vi "SteuerungWaermepumpe - 10.0117_ohne Keithley.vi"() -> ()   [LabVIEW 2015]
uses:
  <vilib>/DAQmx/read.llb/DAQmx Read (Analog 1D Wfm NChan NSamp).vi
  <vilib>/DAQmx/write.llb/DAQmx Write (Analog 1D Wfm NChan 1Samp).vi
  <vilib>/MakerHub/LINX/Public/Peripherals/Digital/Digital Write N Chans.vi
  <vilib>/MakerHub/LINX/Private/Local IO/LinxDigitalWrite.vi
  <vilib>/MakerHub/LINX/Public/Utilities/Check Channel.vi
  <vilib>/MakerHub/LINX/Private/Utilties/Generate Error.vi
  <vilib>/DAQmx/miscellaneous.llb/DAQmx Fill In Error Info.vi
  <vilib>/Utility/file.llb/Read Delimited Spreadsheet (DBL).vi
  <vilib>/MakerHub/LINX/LMH-LINX.lvlib
panel:
  out "Abscheider":cluster{dbl, dbl, dbl}(slide) scale=0.0..1.3
  in  "Rampe":bool=TRUE
  in  "Rampe rpm/s":dbl=1.0 min=1.0 max=100.0 step=1.0
  out "Rampe IW":dbl
  in  "reinitialize HD":bool
  in  "reinitialize Pumpe":bool
  out "ist an!":string
  in  "zusätzlicher Druck":dbl
  in  "PI05 SW":dbl format="%.2f"
  out "p_liq_mittel":dbl
  out "p_liq":dbl
  out "Schleifendauer":dbl format="%.5f"
  out "Mittelwert 2":dbl
  in  "Mittelwert HD":bool
  in  "Mittelwert Pumpe":bool
  out "Mittelwert":dbl
  in  "Xi / p_liq berechnung an":bool
  out "xi_r":dbl
  in  "Regler Senke":bool
  in  "reinitialize Senke":bool
  in  "TI35 SW":dbl=43.0 format="%.2f"
  in  "Drehzahl Bestätigung":bool
  in  "Drehzahl SW":dbl=1000.0 min=500.0 max=3000.0 step=1.0 format="%#_4g"
  out "Check":dbl format="%#_13g"
  in  "Regler Hochdruck":bool
  in  "PID Regelung Pumpe":bool
  in  "SW TI39":dbl
  out "Array":bool[](array[boolean])
  in  "LEDs 2":bool[](array[boolean])
  in  "Regelung HK":bool
  in  "RV 30 zu":bool
  in  "RV 30 auf":bool
  out "FI_Oel":dbl
  in  "RV 33":dbl(slide) scale=-1.0..1.0
  in  "tag":string
  out "Pumpenwerte":dbl[](array[numeric]) format="%.2f"
  out "Speichert!":bool
  out "Historie":string
  in  "Kommentar":string
  out "refnum out":refnum<file>
  in  "Identität!":string(combo)
  in  "Zeit X in Minuten":dbl(slide)=5.0 min=0.0 max=15.0 scale=5.0..15.0
  out "TI 21a Warnungen":dbl
  out "Leistung":dynamicdata(graph)
  out "TI 37":dbl
  in  "Programm stoppen!":bool
  out "%":sgl(slide) scale=0.0..100.0
  out "kalt":bool
  out "warm":bool
  out "?":T1(array[cluster]) {"?" format="%#.4g"; "Konzentration_reich" format="%#.4g"}
  in  "Mit EES vergleichen":bool
  in  "FI13 SW in l/min":dbl=3.0 min=3.0 max=12.0 step=0.10000000149011612
  out "COP_Oel":dbl
  out "Q-Oel kW":dbl format="%_4g"
  in  "Dateiname!":string
  in  "Comment":bool
  in  "Speichern":bool caption="Aktivieren"
  out "ZU     Ventilstellung 33     AUF":dbl(slide) scale=0.0..100.0 scale format="%.2f"
  in  "Regelventil 34":dbl(slide) min=0.0 max=100.0 step=0.009999999776482582 scale=0.0..100.0
  in  "Matlab":bool
  in  "?":T2(tab)
  out "?":dynamicdata(graph)
  out "?":waveform(dbl)(graph)
  out "?":dynamicdata(graph)
  out "PI 12":dbl format="%.2f"
  out "PI 11":dbl format="%.2f"
  out "Dichte":dbl format="%.5g"
  in  "Reset":bool
  out "Betriebszeit":cluster{"second":i32, "minute":i32, "hour":i32}
  out "Temperatur Ölprüfstand":dbl
  out "FI 13 kg/min":dbl
  in  "Messung\nFrequenzwandler":bool
  out "Magnetventil":bool
  out "Fl.Pumpe an":bool
  out "Temperatur Öl":bool
  out "COP":dbl format="%#_13g"
  out "Verdichteraktivität":cluster{"second":i32, "minute":i32, "hour":i32}
  out "Q-Entgaser kW":dbl format="%_4g"
  out "Warnungen":bool[](array[boolean])
  out "Status Komponenten":bool[](array[boolean])
  in  "Pumpen-Auto-Abschalt":bool=TRUE
  out "Q-Resorber kW":dbl format="%_4g"
  out "Stellung Expansionsventil":waveform(dbl)(graph)
  out "FI 35 l/min":dbl format="%#_13g"
  out "FI 38 l/min":dbl format="%#_13g"
  out "FI Oel l/min":dbl format="%#.3g"
  out "LI in l":dbl format="%#_4g"
  out "TI 39":dbl format="%#_3g"
  out "TI 38":dbl format="%#_3g"
  out "TI 36":dbl format="%#_3g"
  out "TI 35":dbl format="%#_3g"
  out "TI 33":dbl format="%#_3g"
  out "TI 32":dbl format="%#_3g"
  out "TI 34":dbl format="%#_3g"
  out "TI 21a":dbl format="%#_3g"
  out "TI 21":dbl format="%#_3g"
  out "TI 20":dbl format="%#_3g"
  out "TI 14a":dbl format="%#_3g"
  out "TI 14":dbl format="%#_3g"
  out "TI 13":dbl format="%#_3g"
  out "TI 12":dbl format="%#_3g"
  out "TI 11":dbl format="%#_3g"
  out "TI 10":dbl format="%#_3g"
  out "TI 09":dbl format="%#_3g"
  out "TI 08":dbl format="%#_3g"
  out "TI 07":dbl format="%#_3g"
  out "TI 06a":dbl format="%#_3g"
  out "TI 06":dbl format="%#_3g"
  out "TI 05":dbl format="%#_3g"
  out "TI 04":dbl format="%#_3g"
  out "TI 22":dbl format="%#_3g"
  out "TI 02":dbl format="%#_3g"
  out "TI 01":dbl format="%#_3g"
  out "Konzentration":dbl format="%#_5g"
  in  "Pumpensteuerung":dbl min=0.0 max=10.0 step=0.009999999776482582 format="%.2g"
  out "PI 08":dbl format="%.2f"
  out "PI 05":dbl format="%#.2f"
  out "PI 02":dbl format="%.2f"
  out "PI 04":dbl format="%.2f"
  out "PDI 8-9":dbl format="%.2f"
  out "PI 14":dbl format="%.2f"
  out "PI 01":dbl format="%.2f"
  out "ZU    Ventilstellung Exp.V     AUF":dbl(slide) scale=0.0..100.0 scale format="%#.1f"
  in  "Exp.V":dbl(slide)=3.0 min=0.0 max=100.0 step=1.0 scale=0.0..100.0 scale format="%#.0f"
  out "ZU    Ventilstellung 14      AUF":dbl(slide) caption="Auf    Ventilstellung 14      Zu" scale=0.0..100.0 scale format="%#.2f"
  in  "Regelventil 36":dbl(slide) min=0.0 max=100.0 step=0.009999999776482582 scale=0.0..100.0 scale format="%#.0f"
  out "ZU  Ventilstellung 35  AUF":dbl(slide) scale=0.0..100.0 scale format="%.2f"
  in  "Regelventil 35":dbl(slide)=100.0 min=0.0 max=100.0 step=0.009999999776482582 scale=0.0..100.0 scale format="%#.3g"
  out "ZU     Ventilstellung 39     AUF":dbl(slide) scale=0.0..100.0 scale format="%.2f"
  in  "Regelventil 39":dbl(slide)=100.0 min=0.0 max=100.0 step=0.009999999776482582 scale=0.0..100.0
  out "FI 13 l/min":dbl format="%.2f"
  out "FI 07 l/min":dbl format="%.2f"
  out "LI in m":dbl format="%.2f"
  out "PDI 5-6":dbl format="%.4f"
  out "PI 07":dbl format="%.2f"
  out "Druckverhältnis":dbl
  out "Drehzahl":dbl
  out "Drehmoment":dbl
  out "Frequenz":dbl
  out "Leistung":dbl
  out "Durchfluss":waveform(dbl)[](graph)
  in  "Tab Control Temperaturen":T3(tab)
  out "Temperatur Reich":waveform(dbl)[](graph)
  out "Temperatur Arm":waveform(dbl)[](graph)
  out "Temperatur Öl":waveform(dbl)[](graph)
  out "Temperatur Senke/Quelle":waveform(dbl)[](graph)
  out "Druck":waveform(dbl)[](graph)
  out "Druckzustand":bool caption="Zu viel Druck !!!"
  # "Öltemperatur"
  # "Resorber"
  # "Entgaser"
  # "Druckverhältnis"
  # "ExpV"
  # "Verdichter an"
  # "iWÜ"
  # "Magnetventil"
  # "RV 39"
  # "RV 35"
  # "RV 33"
  # "RV 34"
  # "Pumpe an"
  # "Ölabscheider"
  # "2"
  # "1"
  # "RV 30"
  # "Verdichter"
  # "Pumpe"
  # "Leistung"
  # "kW"
  # "Speed"
  # "rpm"
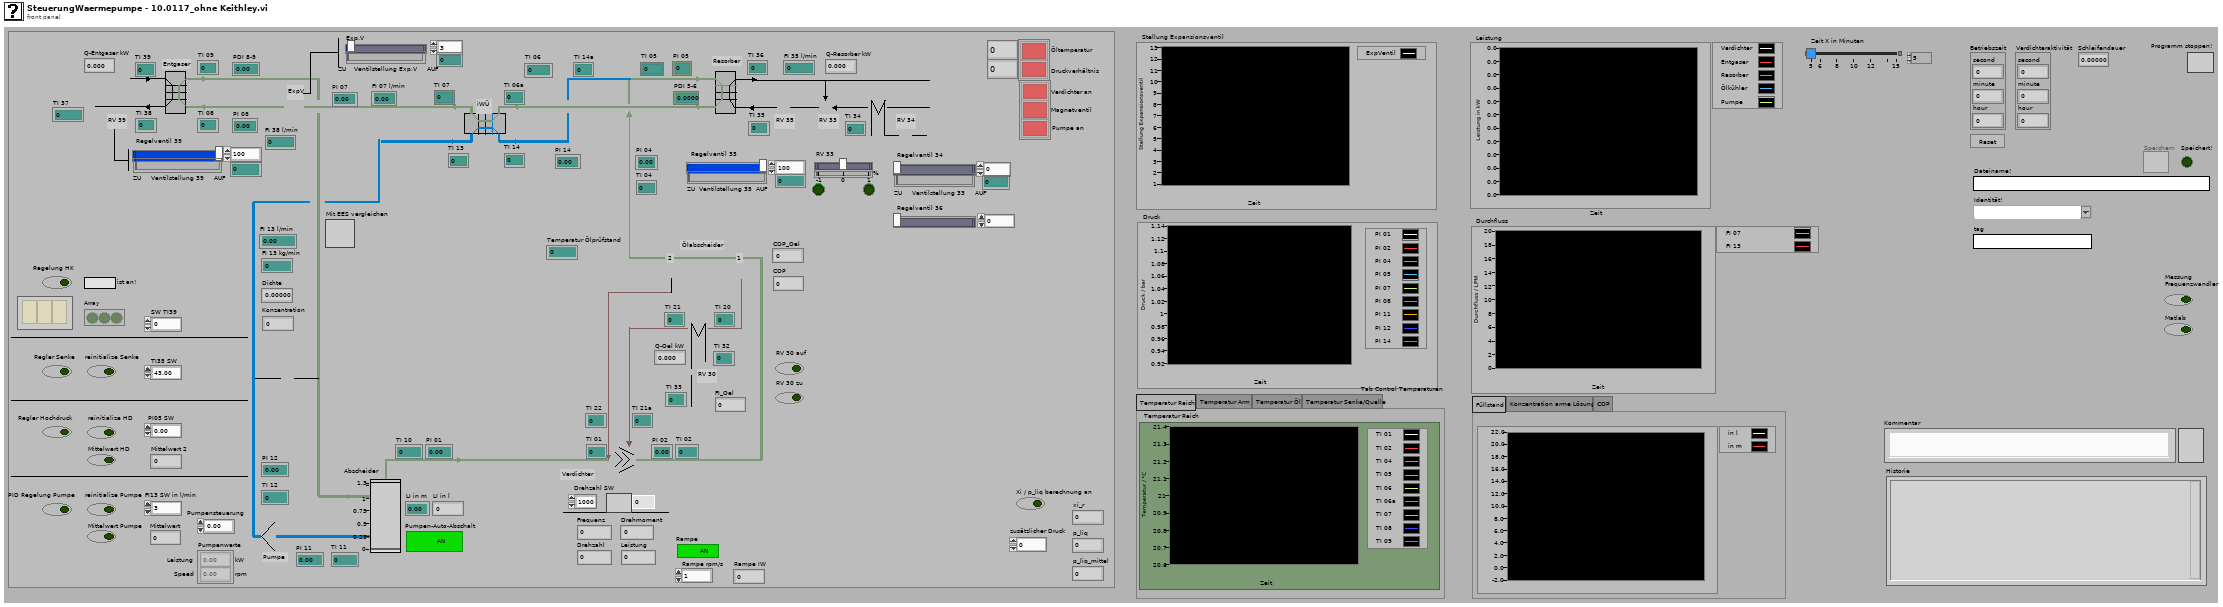
[diagram p1: front panel]
types:
  T1 = cluster{dbl, "Konzentration_reich":dbl, "String":string, bool}[]
  T2 = enum32{"Füllstand", "Konzentration arme Lösung", "COP"}
  T3 = enum32{"Temperatur Reich", "Temperatur Arm", "Temperatur Öl", "Temperatur Senke/Quelle"}
  T4 = enum8{"Enabled", "Disabled", "Disabled and Grayed Out"}
  T5 = typedef "LMH-LINX.lvlib/LINX Ref.ctl" = cluster{"IO":T6, "Interface":T7, "LINX Device Config":T8}
  T6 = typedef "LMH-LINX.lvlib/Platform.ctl" = enum16{"Remote", "Local"}
  T7 = typedef "LMH-LINX.lvlib/Interface.ctl" = enum16{"Serial", "TCP"}
  T8 = typedef "LMH-LINX.lvlib/Device.lvlib/LINX Device Config.ctl" = cluster{"Interface":T7, "COM Port":refnum<visa-resource-name>, "TCP Configuration":T9, "Device Family":u8, "Device ID":u8, "Device Name":string, "TCP Ref":refnum<k5>, "Channels":T10}
  T9 = typedef "LMH-LINX.lvlib/Device.lvlib/TCP Config.ctl" = cluster{"IP Address":string, "Port":u16}
  T10 = typedef "LMH-LINX.lvlib/Channels.ctl" = cluster{"DI":u8[], "DO":u8[], "AI":u8[], "AO":u8[], "PWM":u8[], "QE":u8[], "UART":u8[], "I2C 2":u8[], "SPI":u8[], "CAN":u8[], "Servo":u8[], "AI Ref (V)":dbl, "AI Resolution (Bits)":u8, "AO Ref (V)":dbl, "AO Resolution (Bits)":u8}
  T11 = enum16{"open", "replace", "create", "open or create", "replace or create", "replace or create with confirmation"}
  T12 = cluster{"Array[0]":dbl, "Array[1]":dbl, "Array[2]":dbl}
  T13 = cluster{"Array[0]":sgl, "Array[1]":sgl, "Array[2]":sgl}
  T14 = cluster{"Numeric":dbl, "Konzentration_reich":dbl, "String":string, bool}[]
  T15 = typedef "LVDateTimeRec.ctl" = cluster{"fractional second":dbl, "second":i32, "minute":i32, "hour":i32, "day of month":i32, "month":i32, "year":i32, "day of week":i32, "day of year":i32, "DST":i32}
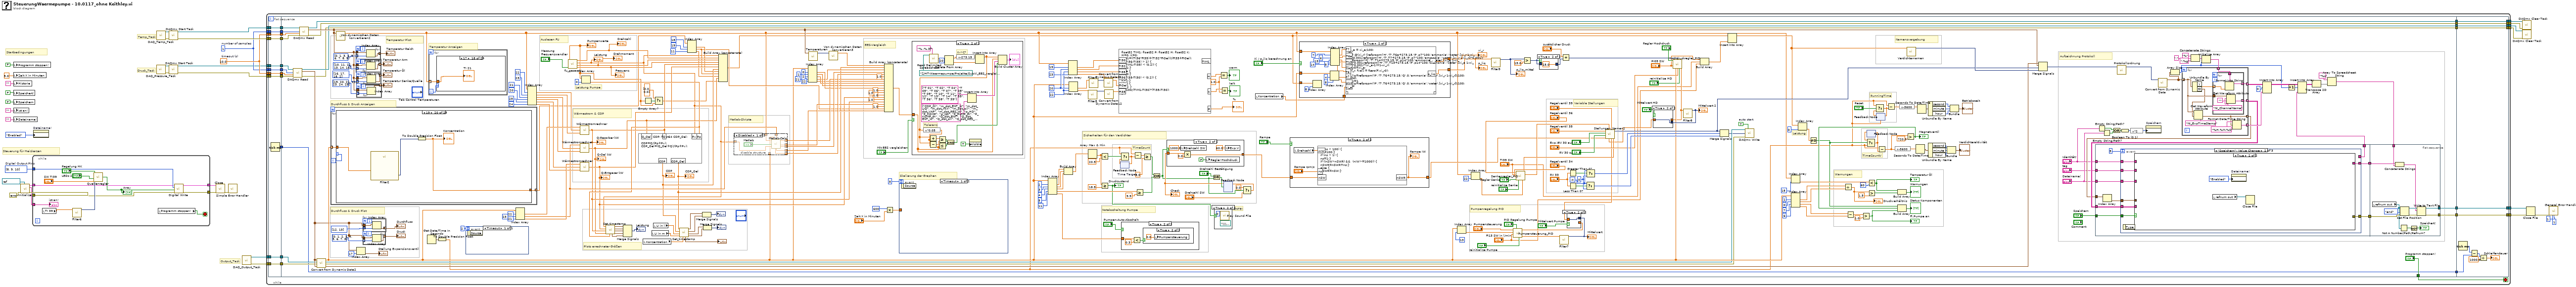
[diagram p0: block diagram]
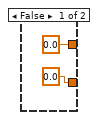
[diagram p8: hidden frame]
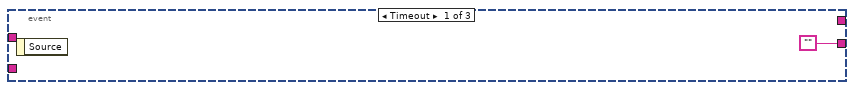
[diagram p10: hidden frame]
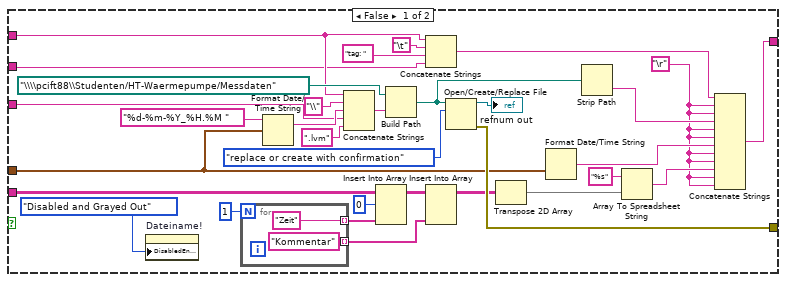
[diagram p11: hidden frame]
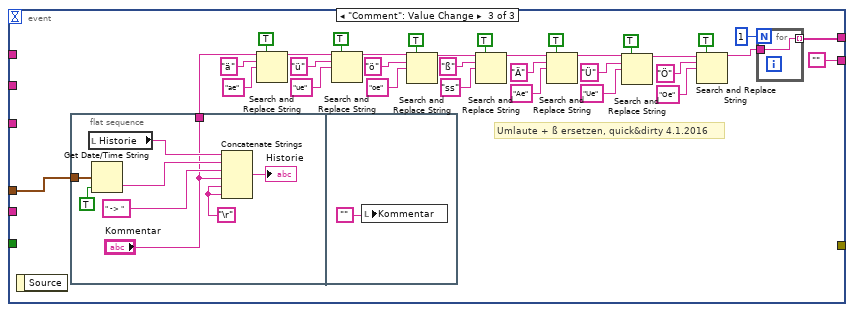
[diagram p12: hidden frame]
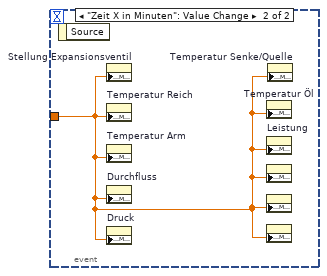
[diagram p13: hidden frame]
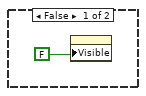
[diagram p14: hidden frame]
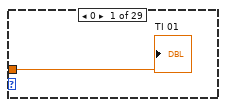
[diagram p17: hidden frame]
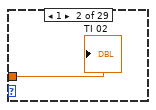
[diagram p18: hidden frame]
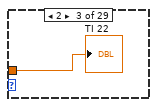
[diagram p19: hidden frame]
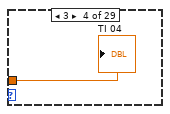
[diagram p20: hidden frame]
diagram:
  w10 = 10.0  # timeout (s)
  w9 = 1  # number of samples
  w22 = i32[] [8, 9, 10]  # Digital Output PIns
  # "Output_Task"
  # "Druck_Task"
  # "Temp_Task"
  # "Steuerung für Heizkerzen"
  # "Startbedingungen"
  n1 = local write "Programm stoppen!"(FALSE ("Programm stoppen!")) -> ()
  n2 = local write "Zeit X in Minuten"(5.0 ("Zeit X in Minuten")) -> ()
  n3 = local write "Historie"("") -> ()
  n4 = local write "Speichert!"(FALSE ("Speichert!")) -> ()
  n5 = local write "Speichern"(FALSE ("Speichern")) -> ()
  n6 = local write "ist an!"("") -> ()
  n7 = local write "Dateiname!"("") -> ()
  n8 = call <vilib>:"Initialize.vi"("Serial Port"=refnum<visa-resource-name> "COM4", "Error In"=errorcluster {"status"=FALSE, "code"=0, "source"=""}) -> ("Error Out"=w23:errorcluster, "Device Name"=w20:string, "LINX Resource"=w26:T5)  [unwired: 7 in]
  n9 = while {
    tunnel: w26 -> [w41]
    tunnel: [w51] -> w25
    tunnel: [w50] -> w24
    tunnel: w23 -> [w40]
    tunnel: w22 -> [w49]
    tunnel: w20 -> [w39]
    stop <- w48 stop-if-true
    n10 = local read "TI 39"() -> (w42:dbl)
    n11 = call "Filter6"("Signal"=w42) -> ("Filtered Signal"=w43:dynamicdata)  [unwired: 9 in, 1 out]
    n12 = call "Quellenregler.vi"("Regelung Quelle"="Regelung HK", "TI 38 IW °C"=w43, "LEDs"="LEDs 2", "TI 38 SW °C"="SW TI39") -> ("Kerzen von Regler"=w45:bool[])  [unwired: 3 in, 1 out]
    "Array" <- w45
    n13 = local read "Programm stoppen!"() -> (w48:bool)
    n14 = call-poly <vilib>:"Digital Write.vi"("Error In"=w40, "Values"=w45, "DO Channels"=w49, "LINX Resource"=w41) -> ("Error Out"=w50:errorcluster, "LINX Resource"=w51:T5)  [unwired: 6 in]
    "ist an!" <- w39
  }
  n15 = property on="Dateiname!" class="Str"("DisabledEnum"=T4."Enabled" ("Disabled")) -> ()  [unwired: 2 in, 2 out]
  n16 = call "DAQ_Pressure_Task.vi"() -> ("error out"=w14:errorcluster, "task out"=w15:refnum<k21>)  [unwired: 10 in]
  n17 = call "DAQ_Temp_Task.vi"() -> ("error out"=w16:errorcluster, "task out"=w17:refnum<k21>)  [unwired: 10 in]
  n18 = call <vilib>:"DAQmx Start Task.vi"("task/channels in"=w15, "error in"=w14) -> ("task out"=w8:refnum<k21>, "error out"=w11:errorcluster)  [unwired: 12 in]
  n19 = call <vilib>:"DAQmx Start Task.vi"("task/channels in"=w17, "error in"=w16) -> ("task out"=w12:refnum<k21>, "error out"=w13:errorcluster)  [unwired: 12 in]
  n20 = call <vilib>:"Close.vi"("Error In"=w24, "LINX Resource"=w25) -> ("Error Out"=w27:errorcluster)  [unwired: 9 in]
  n21 = call <vilib>:"Simple Error Handler.vi"("error in (no error)"=w27) -> ()  [unwired: 4 in, 5 out]
  n22 = call "DAQ_Output_Task.vi"() -> ("error out"=w2:errorcluster, "task out"=w3:refnum<k21>)  [unwired: 10 in]
  n23 = while {
    tunnel: [w86] -> w32
    tunnel: [w85] -> w31
    tunnel: w13 -> [w79]
    tunnel: w10 -> [w77]
    tunnel: w12 -> [w74]
    tunnel: w9 -> [w72]
    tunnel: w11 -> [w70]
    tunnel: w10 -> [w69]
    tunnel: w9 -> [w67]
    tunnel: w8 -> [w65]
    tunnel: [w61] -> w7
    tunnel: [w60] -> w6
    tunnel: [w58] -> w5
    tunnel: [w56] -> w4
    tunnel: w3 -> [w55]
    tunnel: w2 -> [w52]
    stop <- w84 stop-if-true
    n24 = flat-sequence {
      tunnel: [w97] -> w80
      tunnel: w79 -> [w96]
      tunnel: [w96] -> w78
      tunnel: w77 -> [w95]
      tunnel: [w95] -> w76
      tunnel: w74 -> [w94]
      tunnel: [w94] -> w75
      tunnel: [w93] -> w73
      tunnel: w72 -> [w93]
      tunnel: [w92] -> w71
      tunnel: w70 -> [w92]
      tunnel: w69 -> [w91]
      tunnel: [w91] -> w68
      tunnel: w67 -> [w90]
      tunnel: [w90] -> w66
      tunnel: w65 -> [w89]
      tunnel: [w89] -> w64
      tunnel: w55 -> [w88]
      tunnel: [w88] -> w54
      tunnel: [w87] -> w53
      tunnel: w52 -> [w87]
      tunnel: ["Programm stoppen!"] -> w84
      tunnel: [w313] -> w83
      tunnel: [w312] -> w82
      tunnel: [w116] -> w81
      tunnel: w80 -> [w116]
      tunnel: w78 -> [w153]
      tunnel: w76 -> [w152]
      tunnel: w75 -> [w151]
      tunnel: w73 -> [w150]
      tunnel: w71 -> [w149]
      tunnel: w68 -> [w148]
      tunnel: w66 -> [w147]
      tunnel: w64 -> [w146]
      tunnel: [w145] -> w63
      tunnel: [w144] -> w62
      tunnel: [w143] -> w59
      tunnel: [w142] -> w57
      tunnel: w54 -> [w140]
      tunnel: w53 -> [w139]
      tunnel: [w725] -> w85
      tunnel: [w726] -> w86
      tunnel: w83 -> [w726]
      tunnel: w82 -> [w725]
      tunnel: w81 -> [w723]
      tunnel: w63 -> [w718]
      tunnel: w62 -> [w719]
      tunnel: [w719] -> w61
      tunnel: [w718] -> w60
      tunnel: w59 -> [w717]
      tunnel: [w717] -> w58
      tunnel: w57 -> [w716]
      tunnel: [w716] -> w56
      frame #0 {
        n25 = Tick Count (ms)() -> (millisecond timer value=w97:u32)
      }
      frame #1 {
        w118 = 8.0  # Time Target
        w141 = TRUE  # auto start
        w333 = sgl 1.0
        w346 = 22
        w351 = 20
        w377 = -4
        w378 = 0
        # "RunningTime"
        # "TimeCountV"
        # "TimeCount"
        # "ENTE!"
        # "Sicherheiten für den Verdichter"
        # "Pumpenregelung PID"
        # "Skalierung der Graphen"
        # "Leistung Pumpe"
        # "Leistung"
        # "Durchfluss & Druck Anzeigen"
        # "Temperatur Anzeigen"
        # "Plots errechneter Größen"
        # "EES-Vergleich"
        # "Matlab-Skripte"
        # "Warnungen"
        # "Namensvergebung"
        # "Wärmestrom & COP"
        # "Notabschaltung Pumpe"
        # "Auslesen FU"
        # "Durchfluss & Druck Plot"
        # "Temperatur Plot"
        # "Aufzeichnung Protokoll"
        # "Variable Stellungen"
        n26 = call-poly <vilib>:"DAQmx Read.vi"("task/channels in"=w146, "number of samples per channel"=w147, "timeout"=w148, "error in"=w149) -> ("task out"=w145:refnum<k21>, "data"=w155:waveform(dbl)[], "error out"=w142:errorcluster)  [unwired: 9 in]
        n27 = call-poly <vilib>:"DAQmx Read.vi"("task/channels in"=w151, "number of samples per channel"=w150, "timeout"=w152, "error in"=w153) -> ("task out"=w144:refnum<k21>, "data"=w154:waveform(dbl)[], "error out"=w143:errorcluster)  [unwired: 9 in]
        n28 = call "Convert from Dynamic Data2"("Dynamic Data Type"=w155) -> ("Array"=w160:dbl[])  [unwired: 3 in]
        n29 = for {
          tunnel: w160 -> [w664] mode=indexing
          tunnel: [w663] -> w165 mode=indexing
          i -> [w665]
          n30 = case shown="19" w665 {
            tunnel: w664 -> [w666 w667 w668 w669 w670 w671 w672 w673 w674 w675 w676 w685 w697 w700 w701 w702 w703 w704 w707 w711 w712 w713 w714 w715 _]
            tunnel: [_ _ _ _ _ _ _ _ _ _ _ w677 _ _ _ _ _ _ w705 w709 _ _ _ _ _] -> w663
            frame 0 {
              "PI 01" <- w666
            }
            frame 1 {
              "PI 02" <- w667
            }
            frame 2 {
              "PI 04" <- w668
            }
            frame 3 {
              "PI 05" <- w669
            }
            frame 4 {
              "PI 07" <- w670
            }
            frame 5 {
              "PI 08" <- w671
            }
            frame 6 {
              "PI 11" <- w672
            }
            frame 7 {
              "PI 12" <- w673
            }
            frame 8 {
              "PI 14" <- w674
            }
            frame 9 {
              "PDI 5-6" <- w675
            }
            frame 10 {
              "PDI 8-9" <- w676
            }
            frame 11 {
              n31 = call "Filter3"("Signal"=w685) -> ("Filtered Signal"=w683:dynamicdata)  [unwired: 9 in, 1 out]
              n32 = Greater?(x=w685, y=0.3) -> (0:w680:bool)
              n33 = case shown="False" w680 {
                tunnel: w685 -> [_ w696]
                tunnel: [0.0 w696] -> w688
                frame False {
                }
                frame True {
                }
              }
              n34 = call "Convert from Dynamic Data6"("Dynamic Data Type"=w683) -> ("Scalar"=w682:dbl)  [unwired: 3 in]
              n35 = Multiply(x=w682, y=10.0) -> (x*y=w684:dbl)
              n36 = Greater?(x=w685, y=0.4) -> (0:w681:bool)
              n37 = formula code="float64 y; float64 Vu; /*Vu: Volumen schmaler Zylinder+Fuellstandsmesser*/\nVu=10;  /* 10 Liter */\n\nif (x<=10.25) \ny=(x-1)*pi*(0.536**2+0.32**2);\nelse\ny=Vu+(x-10.25)*pi*(1.584**2+0.32**2);"("x"=w684) -> ("y"=w677:dbl)
              "LI in l" <- w677
              n38 = case shown="False" w681 {
                tunnel: w685 -> [_ w694]
                tunnel: [0.0 w694] -> w687
                frame False {
                }
                frame True {
                }
              }
              n39 = Merge Signals(w685, w688, w687) -> (w689:dynamicdata)
              n40 = call "Convert from Dynamic Data3"("Dynamic Data Type"=w689) -> ("Array"=w692:dbl[])  [unwired: 3 in]
              n41 = Array To Cluster(array=w692) -> (cluster=w679:T12)
              n42 = To Single Precision Float(number=w679) -> (single precision float=→"Abscheider":T13)
              "LI in m" <- w685
            }
            frame 12 {
              "FI 07 l/min" <- w697
            }
            frame 13 {
              n43 = local read "Dichte"() -> (w699:dbl)
              n44 = Multiply(x=w700, y=w699) -> (x*y=→"FI 13 kg/min":dbl)
              "FI 13 l/min" <- w700
            }
            frame 14 {
              "ZU     Ventilstellung 39     AUF" <- w701
              "ZU     Ventilstellung 33     AUF" <- w701
            }
            frame 15 {
              "ZU  Ventilstellung 35  AUF" <- w702
            }
            frame 16 {
              # "RV14 ist entfernt"
              "ZU    Ventilstellung 14      AUF" <- w703
            }
            frame 17 {
              "ZU    Ventilstellung Exp.V     AUF" <- w704
            }
            frame 18 {
              n45 = call "Filter"("Signal"=w707) -> ("Filtered Signal"=w706:dynamicdata)  [unwired: 9 in, 1 out]
              n46 = call "Convert from Dynamic Data4"("Dynamic Data Type"=w706) -> ("Scalar"=w708:dbl)  [unwired: 3 in]
              n47 = formula code="float64 D;\nD=9.375*StromDichte+0.7125;\nD=floor(D*100000)/100000;"("StromDichte"=w708) -> ("D"=w705:dbl)
              "Dichte" <- w705
            }
            frame 19 {
              n48 = call "Filter2"("Signal"=w711) -> ("Filtered Signal"=w710:dynamicdata)  [unwired: 9 in, 1 out]
              n49 = To Double Precision Float(number=w710) -> (double precision float=w709:dbl)
              "Konzentration" <- w709
            }
            frame 20 {
              "FI Oel l/min" <- w712
            }
            frame 21 {
              "FI 38 l/min" <- w713
            }
            frame 22 {
              "FI 35 l/min" <- w714
            }
            frame 23 {
              "FI_Oel" <- w715
            }
            frame 24, Default {
            }
          }
        }
        n50 = call "Von dynamischen Daten konvertieren2"("Dynamic Data Type"=w154) -> ("Array"=w101:dbl[])  [unwired: 3 in]
        n51 = for {
          tunnel: i32[] [0, 1, 3, 4, 5, 6, 7, 8, 9] -> [w478] mode=indexing
          tunnel: w154 -> [w477]
          tunnel: [w476] -> w249 mode=indexing
          n52 = Index Array(array=w477, index=w478) -> (element=w476:waveform(dbl))
        }
        "Temperatur Reich" <- w249
        n53 = for {
          tunnel: i32[] [10, 11, 12, 13, 14, 15] -> [w475] mode=indexing
          tunnel: w154 -> [w474]
          tunnel: [w473] -> w250 mode=indexing
          n54 = Index Array(array=w474, index=w475) -> (element=w473:waveform(dbl))
        }
        "Temperatur Arm" <- w250
        n55 = for {
          tunnel: i32[] [16, 17, 18, 2] -> [w472] mode=indexing
          tunnel: w154 -> [w471]
          tunnel: [w470] -> w251 mode=indexing
          n56 = Index Array(array=w471, index=w472) -> (element=w470:waveform(dbl))
        }
        "Temperatur Öl" <- w251
        n57 = Index Array(array=w155, index=17) -> (element=→"Stellung Expansionsventil":waveform(dbl))
        n58 = for {
          tunnel: i32[] [19, 20, 21, 22, 23, 24, 25] -> [w469] mode=indexing
          tunnel: w154 -> [w468]
          tunnel: [w467] -> w252 mode=indexing
          n59 = Index Array(array=w468, index=w469) -> (element=w467:waveform(dbl))
        }
        "Temperatur Senke/Quelle" <- w252
        n60 = for {
          tunnel: [w463] -> w247 mode=indexing
          tunnel: w155 -> [w462]
          tunnel: i32[] [0, 1, 2, 3, 4, 5, 6, 7, 8] -> [w461] mode=indexing
          n61 = Index Array(array=w462, index=w461) -> (element=w463:waveform(dbl))
        }
        "Druck" <- w247
        n62 = for {
          tunnel: [w466] -> w248 mode=indexing
          tunnel: w155 -> [w465]
          tunnel: i32[] [12, 13] -> [w464] mode=indexing
          n63 = Index Array(array=w465, index=w464) -> (element=w466:waveform(dbl))
        }
        "Durchfluss" <- w248
        n64 = Get Date/Time In Seconds() -> (seconds since 1Jan1904=w115:timestamp)
        n65 = for {
          tunnel: w101 -> [w633] mode=indexing
          i -> [w634]
          n66 = case shown="17" w634 {
            tunnel: w633 -> [w635 w636 w637 w638 w639 w640 w641 w642 w643 w644 w645 w646 w647 w648 w649 w650 w651 w652 w653 w654 w655 w656 w657 w658 w659 w660 w661 w662 _]
            frame 0 {
              "TI 01" <- w635
            }
            frame 1 {
              "TI 02" <- w636
            }
            frame 2 {
              "TI 22" <- w637
            }
            frame 3 {
              "TI 04" <- w638
            }
            frame 4 {
              "TI 05" <- w639
            }
            frame 5 {
              "TI 06" <- w640
            }
            frame 6 {
              "TI 06a" <- w641
            }
            frame 7 {
              "TI 07" <- w642
            }
            frame 8 {
              "TI 08" <- w643
            }
            frame 9 {
              "TI 09" <- w644
            }
            frame 10 {
              "TI 10" <- w645
            }
            frame 11 {
              "TI 11" <- w646
            }
            frame 12 {
              "TI 12" <- w647
            }
            frame 13 {
              "TI 13" <- w648
            }
            frame 14 {
              "TI 14" <- w649
            }
            frame 15 {
              "TI 14a" <- w650
            }
            frame 16 {
              "TI 20" <- w651
            }
            frame 17 {
              "TI 21" <- w652
            }
            frame 18 {
              "TI 21a" <- w653
              "TI 21a Warnungen" <- w653
            }
            frame 19 {
              # "Check T_Heater"
              "TI 34" <- w654
            }
            frame 20 {
              "TI 32" <- w655
            }
            frame 21 {
              "TI 33" <- w656
            }
            frame 22 {
              "TI 35" <- w657
            }
            frame 23 {
              "TI 36" <- w658
            }
            frame 24 {
              "TI 38" <- w659
            }
            frame 25 {
              "TI 39" <- w660
            }
            frame 26 {
              "Temperatur Ölprüfstand" <- w661
            }
            frame 27 {
              "TI 37" <- w662
            }
            frame 28, Default {
            }
          }
        }
        n67 = To Double Precision Float(number=w115) -> (double precision float=w103:dbl)
        n68 = event shown="[0] Timeout" {
          selector: _ -> [_]
          dyn-events: _ -> [_]
          timeout: 2 -> [_]
          event Timeout {
            n69 = event-data() -> ()  [unwired: 1 in, 1 out]
          }
        }
        n70 = Index Array(array=w160, index #1=22 ("index"), index #2=23 ("index"), index #3=21 ("index")) -> (element #1=w282:dbl, element #2=w258:dbl, element #3=w281:dbl)
        n71 = Index Array(array=w101, index #1=22 ("index"), index #2=23 ("index"), index #3=21 ("index"), index #4=20 ("index"), index #5=25 ("index"), index #6=24 ("index")) -> (element #1=w280:dbl, element #2=w279:dbl, element #3=w278:dbl, element #4=w277:dbl, element #5=w276:dbl, element #6=w275:dbl)
        n72 = call "fu_gesamt.vi"("Boolean"="Messung\nFrequenzwandler") -> ("Frequenz"=w270:dbl, "Drehmoment"=w271:dbl, "Leistung"=w126:dbl, "Drehzahl"=w272:dbl, "Scaled"=w128:dbl[])  [unwired: 6 in]
        "Leistung" <- w126
        "Frequenz" <- w270
        "Drehmoment" <- w271
        "Drehzahl" <- w272
        "Pumpenwerte" <- w128
        n73 = call "Wärmestromrechner.vi"("Taus"=w279, "Tein"=w280, "Massenstrom"=w282) -> ("Wärmestrom Q"=w179:dbl)  [unwired: 2 in]
        "Q-Resorber kW" <- w179
        n74 = call "Wärmestromrechner.vi"("Taus"=w277, "Tein"=w278, "Massenstrom"=w258) -> ("Wärmestrom Q"=w166:dbl)  [unwired: 2 in]
        "Q-Oel kW" <- w166
        n75 = call "Wärmestromrechner.vi"("Taus"=w275, "Tein"=w276, "Massenstrom"=w281) -> ("Wärmestrom Q"=w178:dbl)  [unwired: 2 in]
        "Q-Entgaser kW" <- w178
        n76 = Index Array(array=w128, index=0) -> (element=w180:dbl)
        n77 = call "Set_timestamp.vi"("Eingang 5"=w180, "Eingang 4"=w166, "Eingang 3"=w179, "Eingang 2"=w178, "Eingang"=w126) -> ("Ausgang 4"=w176:waveform(dbl), "Ausgang 3"=w175:waveform(dbl), "Ausgang 2"=w174:waveform(dbl), "Ausgang"=w173:waveform(dbl), "Ausgang 5"=w177:waveform(dbl))  [unwired: 2 in]
        n78 = Merge Signals(w173, w174, w175, w176, w177) -> (→"Leistung":dynamicdata)
        n79 = formula code="float64 COP; float64 COP_Oel;\n\nCOP=Q/(Pp+Pv);\nCOP_Oel=(Q_Oel+Q)/(Pp+Pv);"("Pv"=w126, "Q"=w179, "Pp"=w180, "Q_Oel"=w166) -> ("COP"=w188:dbl, "COP_Oel"=w187:dbl)
        "COP" <- w188
        "COP_Oel" <- w187
        n80 = local read "Konzentration"() -> (w192:dbl)
        n81 = Empty Array?(array=w128) -> (empty?=w130:bool)
        n82 = local read "LI in m"() -> (w190:dbl)
        n83 = local read "LI in l"() -> (w189:dbl)
        n84 = Select(t=dbl[] [0.0, 0.0], s=w130, f=w128) -> (s? t:f=w127:dbl[])
        n85 = call "Set_timestamp.vi"("Eingang 5"=w192, "Eingang 4"=w190, "Eingang 3"=w189, "Eingang 2"=w188, "Eingang"=w187) -> ("Ausgang 4"=w185:waveform(dbl), "Ausgang 3"=w184:waveform(dbl), "Ausgang 2"=w182:waveform(dbl), "Ausgang"=w181:waveform(dbl), "Ausgang 5"=→"?":waveform(dbl))  [unwired: 2 in]
        n86 = Index Array(array=w165, index #1=18 ("index"), index #2=19 ("index"), index #3=11 ("index")) -> (element #1=w167:dbl, element #2=w164:dbl, element #3=w168:dbl)
        n87 = Merge Signals(w181, w182) -> (→"?":dynamicdata)
        n88 = Merge Signals(w184, w185) -> (→"?":dynamicdata)
        n89 = Build Array (concatenate)(w126, w272, w271, w270, w179, w178, w188, w167, w164, w168, w166, w127) -> (w100:dbl[])
        n90 = disable-structure shown="Disabled" {
          disable-tunnel: [w423 _] -> w374
          disable-tunnel: [w422 _] -> w363
          disable-tunnel: [w421 _] -> w352
          disable-tunnel: [w420 _] -> w274
          disable-tunnel: [w419 _] -> w269
          disable-tunnel: w258 -> [w418 _]
          disable-tunnel: w126 -> [w417 _]
          disable-tunnel: w160 -> [w416 _]
          disable-tunnel: w101 -> [w415 _]
          frame Disabled {
            n91 = call "Matlab-Calc.vi"("Temp-Array"=w415, "Matlab?"="Matlab", "Leistung"=w417, "Druck-Array"=w416, "FI Öl"=w418) -> ("m_reich [g/s]"=w422:dbl, "Konzentration_reich"=w419:dbl, "m_arm [g/s]"=w423:dbl, "Dampfmassenstrom [g/s]"=w420:dbl, "Dampfmassenanteil"=w421:dbl)  [unwired: 3 in, 7 out]
          }
          frame Enabled {
          }
        }
        n92 = Index Array(array=w160, index #1=0 ("index"), index #2=1 ("index"), index #3=2 ("index"), index #4=21 ("index"), index #5=22 ("index")) -> (element #1=w357:dbl, element #2=w358:dbl, element #3=w359:dbl, element #4=w356:dbl, element #5=w354:dbl)
        n93 = call "Temperaturen"("Signals"=w154) -> ("Signal Out"=w364:dynamicdata)  [unwired: 9 in, 1 out]
        n94 = call "Von dynamischen Daten konvertieren3"("Dynamic Data Type"=w364) -> ("Array"=w365:dbl[])  [unwired: 3 in]
        n95 = Build Array (concatenate)(w365, w187, w356, w374, w363, 1.0 ("element"), w274, w354, w359, w358, w357, 1.0 ("element"), 1.0 ("element"), 1.0 ("element"), w178, 1.0 ("element"), w179, w352, 1.0 ("element"), w164, w269) -> (w366:dbl[])
        n96 = Multiply(x=600, y="Zeit X in Minuten") -> (x*y=w325:dbl)
        n97 = event shown="[0] Timeout" {
          selector: _ -> [_ _]
          dyn-events: _ -> [_ _]
          timeout: 5 -> [_ _]
          tunnel: w325 -> [_ w607]
          event Timeout {
            n98 = event-data() -> ()  [unwired: 1 in, 1 out]
          }
          event "Zeit X in Minuten": Value Change {
            n99 = event-data() -> ()  [unwired: 1 in, 1 out]
            n100 = property on="Stellung Expansionsventil" class="WFChart (strict)"("XScale.Maximum"=w607) -> ()  [unwired: 2 in, 2 out]
            n101 = property on="Temperatur Reich" class="WFChart (strict)"("XScale.Maximum"=w607) -> ()  [unwired: 2 in, 2 out]
            n102 = property on="Temperatur Arm" class="WFChart (strict)"("XScale.Maximum"=w607) -> ()  [unwired: 2 in, 2 out]
            n103 = property on="Durchfluss" class="WFChart (strict)"("XScale.Maximum"=w607) -> ()  [unwired: 2 in, 2 out]
            n104 = property on="Druck" class="WFChart (strict)"("XScale.Maximum"=w607) -> ()  [unwired: 2 in, 2 out]
            n105 = property on="Temperatur Öl" class="WFChart (strict)"("XScale.Maximum"=w607) -> ()  [unwired: 2 in, 2 out]
            n106 = property on="Leistung" class="WFChart (strict)"("XScale.Maximum"=w607) -> ()  [unwired: 2 in, 2 out]
            n107 = property class="WFChart (strict)"("XScale.Maximum"=w607) -> ()  [unwired: 2 in, 2 out]
            n108 = property class="WFChart (strict)"("XScale.Maximum"=w607) -> ()  [unwired: 2 in, 2 out]
            n109 = property class="WFChart (strict)"("XScale.Maximum"=w607) -> ()  [unwired: 2 in, 2 out]
            n110 = property on="Temperatur Senke/Quelle" class="WFChart (strict)"("XScale.Maximum"=w607) -> ()  [unwired: 2 in, 2 out]
          }
        }
        n111 = case shown="True" "Mit EES vergleichen" {
          tunnel: w366 -> [_ w609]
          frame False {
            n112 = property class="Arr (strict)"("Visible"=FALSE) -> ()  [unwired: 2 in, 2 out]
          }
          frame True {
            # "K->C°"
            # "Toleranz"
            n113 = call-poly <vilib>:"Read Delimited Spreadsheet.vi"("file path (dialog if empty)"=path "Z:/HT-Waermepumpe/Projekte/SubVi_EES_vergleich/test.txt", "format (%.3f)"="%,;%.3f") -> ("first row"=w616:dbl[])  [unwired: 8 in, 5 out]
            n114 = Delete From Array(array=w616, length=20) -> (deleted portion=w612:dbl[], array with subset deleted=w614:dbl[])  [unwired: 1 in]
            n115 = expression code="x-273.15"(w614) -> (w613:dbl[])
            n116 = Insert Into Array(array=string[] ["T 01", "T 02", "T 04", "T 05", "T 06", "T 07", "T 08", "T 09", "T 10", "T 11", "T 12", "T 13", "T 14", "T 35", "T 36", "T 38", "T 39"] ("Array"), new element=string[] ["COP_Öl", "m_dot_ENT_W", "m_dot_LIQ", "m_dot_MIX", "m_dot_oil", "m_dot_VAP", "m_dot_RES_W", "p_HD", "P_KOMP", "p_ND", "P_PUMP_th", "P_KOMP_th", "Q_dot_ENT", "Q_dot_ENT_W", "Q_dot_oil", "Q_dot_RES_W", "q_geg", "Q_dot_RES", "xi_LIQ", "xi_MIX"] ("Array")) -> (w623:string[])  [unwired: 1 in]
            n117 = property class="Arr (strict)"("Visible"=TRUE) -> ()  [unwired: 2 in, 2 out]
            n118 = Insert Into Array(array=w613, new element=w612) -> (w610:dbl[])  [unwired: 1 in]
            n119 = expression code="x*0.05"(w610) -> (w611:dbl[])
            n120 = Add(x=w610, y=w611) -> (x+y=w619:dbl[])
            n121 = Subtract(x=w610, y=w611) -> (x-y=w618:dbl[])
            n122 = Greater Or Equal?(x=w619, y=w609) -> (x >= y?=w620:bool[])
            n123 = Less Or Equal?(x=w618, y=w609) -> (x <= y?=w621:bool[])
            n124 = And(x=w620, y=w621) -> (x .and. y?=w617:bool[])
            n125 = Build Cluster Array(w610, w609, w623, w617) -> (→"?":T14)
          }
        }
        n126 = Index Array(array=w160, index #1=2 ("index"), index #2=3 ("index"), index #3=4, index #4=5, index #5=11 ("index")) -> (element #1=w228:dbl, element #2=w227:dbl, element #3=w226:dbl, element #4=w232:dbl, element #5=w208:dbl)
        n127 = Build Array(w228, w227, w226) -> (w225:dbl[])
        n128 = Index Array(array=w101, index #1=19, index #2=w351, index #3=w346, index #4=23) -> (element #1=w343:dbl, element #2=w342:dbl, element #3=w341:dbl, element #4=w340:dbl)
        n129 = Index Array(array=w160, index #1=w351, index #2=w346) -> (element #1=w349:dbl, element #2=w348:dbl)
        n130 = Array Max & Min(array=w225) -> (min value=w121:dbl)  [unwired: 3 out]
        n131 = call "Filter5"("Signal"=w348) -> ("Filtered Signal"=w344:dynamicdata)  [unwired: 9 in, 1 out]
        n132 = call "Filter4"("Signal"=w349) -> ("Filtered Signal"=w345:dynamicdata)  [unwired: 9 in, 1 out]
        n133 = Less?(x=w121, y=20.5 ("x")) -> (x < y?=w120:bool)
        n134 = Greater Or Equal?(x=w121, y=18.5 ("x")) -> (x >= y?=w98:bool)
        "Druckzustand" <- w98
        n135 = call "Convert from Dynamic Data11"("Dynamic Data Type"=w345) -> ("Scalar"=w339:dbl)  [unwired: 3 in]
        n136 = call "Convert from Dynamic Data12"("Dynamic Data Type"=w344) -> ("Scalar"=w338:dbl)  [unwired: 3 in]
        n137 = formula code="float32 TIM1; float32 P; float32 H; float32 K;\nH=0; K=0;\nTIM1=((TI36*FI35)+(TI32*FIOel))/(FI35+FIOel);\nif((TI36-TI35) > 2) {\nif((TIM1-TI35) < (0.2)) {\nH=1;}\nelse {\nH=0;}\nif((TI35-TI30) < (0.2)) {\nK=1;}\nelse {\nK=0; }\nP=100/(TIM1-TI30)*(TI35-TI30);\n}"("TI30"=w343, "TI32"=w342, "TI35"=w341, "TI36"=w340, "FIOel"=w339, "FI35"=w338) -> ("H"=w337:sgl, "K"=w334:sgl, "P"=→"%":sgl)  [unwired: 1 out]
        n138 = feedback #1() -> (w112:dbl)  [unwired: 1 in]
        n139 = Select(t=w103, s=w120, f=w112) -> (s? t:f=w113:dbl)
        n140 = feedback-in #1(w113) -> ()
        n141 = case shown="True" "Pumpen-Auto-Abschalt" {
          tunnel: w208 -> [_ w630]
          frame False {
          }
          frame True {
            n142 = Less?(x=w630, y=0.3) -> (x < y?=w629:bool)
            n143 = case shown="True" w629 {
              frame False {
              }
              frame True {
                n144 = local write "Pumpensteuerung"(0.0) -> ()
              }
            }
          }
        }
        n145 = Subtract(x=w103, y=w113) -> (x-y=w119:dbl)
        n146 = Greater Or Equal?(x=w232, y=9.9 ("x")) -> (x >= y?=w236:bool)
        n147 = Greater Or Equal?(x=w119, y=w118) -> (x >= y?=w117:bool)
        n148 = Or(x=w117, y=w236) -> (x .or. y?=w218:bool)
        n149 = Or(x="Drehzahl Bestätigung", y=w218) -> (x .or. y?=w220:bool)
        n150 = case shown="True" w98 {
          frame False {
          }
          frame True {
            n151 = call <vilib>:"Play Sound File.vi"("path"=path "\\\\PCIFT88\\Studenten/Niculovic/LV Spielerei/Ente.wav", "device ID"=u32 0) -> ()  [unwired: 8 in, 2 out]
          }
        }
        n152 = Equal?(x=w337, y=w333) -> (x = y?=→"warm":bool)
        n153 = Equal?(x=w334, y=w333) -> (x = y?=→"kalt":bool)
        n154 = feedback #2() -> (w219:dbl)  [unwired: 1 in]
        "Check" <- w219
        n155 = case shown="True" w218 {
          tunnel: w219 -> [w454 w458]
          tunnel: [w454 w459] -> w125
          frame False {
          }
          frame True {
            n156 = local write "Drehzahl SW"(1000.0) -> ()
            n157 = Multiply(x=w458, y=0.0) -> (x*y=w459:dbl)
            n158 = local write "Regler Hochdruck"(FALSE ("Regler Hochdruck")) -> ()
            n159 = local write "Exp.V"(60.0 ("Exp.V")) -> ()
          }
        }
        n160 = Select(t=0.0, s=w218, f="Drehzahl SW") -> (s? t:f=w222:dbl)
        n161 = feedback-in #2(w222, w220) -> ()
        n162 = local read "Konzentration"() -> (w99:dbl)
        n163 = case shown="True" "Rampe" {
          tunnel: [w410 w411] -> w124
          tunnel: w125 -> [w410 w413]
          frame False {
          }
          frame True {
            n164 = local read "Drehzahl"() -> (w412:dbl)
            n165 = formula code="if (ns > 100) {\nns=100;}\nif (ns < 1) {\nns=1;}\nif ((nSW>nSWR) &&  (nIW>=1000)) {\nnSWR=nSWR+ns;}\nelse {\nnSWR=nSW;}"("nSW"=w413, "ns"="Rampe rpm/s", "nIW"=w412) -> ("nSWR"=w411:dbl)
            "Rampe IW" <- w411
          }
        }
        n166 = case shown="True" "Xi / p_liq berechnung an" {
          tunnel: w101 -> [_ w453]
          tunnel: w160 -> [_ w446]
          tunnel: [0.0 w439] -> w210
          tunnel: [0.0 w436] -> w200
          tunnel: w100 -> [_ w434]
          tunnel: w99 -> [_ w433]
          frame False {
          }
          frame True {
            n167 = Index Array(array=w434, index=8) -> ()  [unwired: 1 out]
            n168 = Index Array(array=w446, index #1=4 ("index"), index #2=8 ("index")) -> (element #1=w441:dbl, element #2=w440:dbl)
            n169 = Index Array(array=w453, index #1=7 ("index"), index #2=6 ("index"), index #3=13 ("index"), index #4=14 ("index"), index #5=5 ("index")) -> (element #1=w445:dbl, element #2=w444:dbl, element #3=w443:dbl, element #4=w442:dbl, element #5=w437:dbl)
            n170 = script code="xi_a = xi_a/100;\ntry\nF = @(xi_r) ((refpropm('H','T',T6a+273.15,'P',p7*100,'ammonia','water',[xi_r 1-xi_r])*0.001-refpropm('H','T',T7+273.15,'P',p7*100,'ammonia','water',[xi_r 1-xi_r])*0.001)/(refpropm('H','T',T14+273.15,'P',p14*100,'ammonia','water',[xi_a 1-xi_a])*0.001-refpropm('H','T',T13+273.15,'P',p14*100,'ammonia','water',[xi_a 1-xi_a])*0.001)*(xi_a-1)+1-xi_r);\nxi_r0=xi_a;\n[xi_r, fval] = fzero(F,xi_r0);\n\np_liq=refpropm('P','T',T6+273.15,'Q',0,'ammonia','water',[xi_r 1-xi_r])/100;\ncatch\nxi_r=1\np_liq=refpropm('P','T',T6+273.15,'Q',0,'ammonia','water',[xi_r 1-xi_r])/100;\nend"("T7"=w445, "T6a"=w444, "T13"=w443, "T14"=w442, "xi_a"=w433, "p7"=w441, "p14"=w440, "T6"=w437) -> ("xi_r"=w439:dbl, "p_liq"=w436:dbl)  [unwired: 1 in, 1 out]
          }
        }
        "xi_r" <- w210
        "p_liq" <- w200
        n171 = Index Array(array=w160, index=13) -> (element=w162:dbl)
        n172 = Index Array(array=w101, index=22) -> (element=w135:dbl)
        n173 = call "Filter9"("Signal"=w200) -> ("Filtered Signal"=w198:dynamicdata)  [unwired: 9 in, 1 out]
        "p_liq_mittel" <- w198
        n174 = call "Pumpensteuerung_PID.vi"("reinitialize? (F)"="reinitialize Pumpe", "PID Regelung Pumpe"="PID Regelung Pumpe", "FI13 SW in l/min"="FI13 SW in l/min", "Prozessvariable"=w162, "Pumpensteuerung"="Pumpensteuerung") -> ("upper limit"=w205:dbl)  [unwired: 4 in, 2 out]
        n175 = call "Senkenregler_PID.vi"("Regelventil 36"="Regelventil 36", "Solltemp."="TI35 SW", "Regelventil 34"="Regelventil 34", "Regler Senke"="Regler Senke", "reinitialize?"="reinitialize Senke", "TI_35"=w135) -> ("upper limit 2"=w214:dbl, "upper limit"=w212:dbl)  [unwired: 6 in, 2 out]
        n176 = Greater?(x=w198, y=15.0) -> (0:w197:dynamicdata)
        n177 = case shown="True" w197 {
          tunnel: [w425 15.0 ("y")] -> w196
          tunnel: w197 -> [w425 _]
          frame False {
          }
          frame True {
          }
        }
        n178 = call "Filter7"("Signal"=w205) -> ("Filtered Signal"=w204:dynamicdata)  [unwired: 9 in, 1 out]
        "Mittelwert" <- w204
        n179 = Add(x="zusätzlicher Druck", y=w196) -> (x+y=w195:dynamicdata)
        n180 = case shown="True" "Mittelwert Pumpe" {
          tunnel: w205 -> [w429 _]
          tunnel: [w429 w430] -> w206
          tunnel: w204 -> [_ w430]
          frame False {
          }
          frame True {
          }
        }
        n181 = Greater Than 0?(x="RV 33") -> (x > 0?=w242:bool)
        n182 = Less Than 0?(x="RV 33") -> (x < 0?=w241:bool)
        n183 = Select(t=w377, s=w241, f=w378) -> (s? t:f=w375:i32)
        n184 = Select(t=w377, s=w242, f=w378) -> (s? t:f=w376:i32)
        n185 = call "Hochdruckregler_PID.vi"("Regler Hochdruck"="Regler Hochdruck", "Steuereingang"=w195, "Solldruck"="PI05 SW", "PI05"=w160, "Exp.V"="Exp.V", "reinitialize? (F) in"="reinitialize HD") -> ("upper limit out"=w137:dbl)  [unwired: 7 in, 2 out]
        n186 = call "Filter8"("Signal"=w137) -> ("Filtered Signal"=w201:dynamicdata)  [unwired: 9 in, 1 out]
        "Mittelwert 2" <- w201
        n187 = case shown="True" "Mittelwert HD" {
          tunnel: w137 -> [w427 _]
          tunnel: [w427 w428] -> w202
          tunnel: w201 -> [_ w428]
          frame False {
          }
          frame True {
          }
        }
        n188 = call "Stellungen_Namen2.vi"("Kühlventil"=w214, "Pumpensteuerung"=w206, "Regelventil 39"="Regelventil 39", "Exp.V"=w202, "Regelventil 14"=w212, "Meter"=w124, "zu"="RV 30 zu", "auf"="RV 30 auf", "Regelventil 35"="Regelventil 35") -> ("Dynamic Data"=w273:dynamicdata)  [unwired: 2 in]
        n189 = Build Array("PI05 SW", "TI35 SW", "FI13 SW in l/min") -> (w131:dbl[])
        n190 = Merge Signals(w273, w376, w375) -> (w138:dynamicdata)
        n191 = Insert Into Array(array=w100, new element=w131) -> (w102:dbl[])  [unwired: 1 in]
        n192 = call-poly <vilib>:"DAQmx Write.vi"("task/channels in"=w140, "auto start"=w141, "data"=w138, "error in"=w139) -> ()  [unwired: 9 in, 3 out]
        n193 = Index Array(array=w101, index=18) -> (element=w265:dbl)
        n194 = Index Array(array=w160, index #1=1, index #2=0, index #3=7, index #4=6) -> (element #1=w262:dbl, element #2=w261:dbl, element #3=w260:dbl, element #4=w259:dbl)
        n195 = Index Array(array=w102, index=0) -> (element=w193:dbl)
        n196 = Not Equal To 0?(x=w193) -> (x != 0?=w111:bool)
        n197 = Divide(x=w262, y=w261) -> (x/y=w383:dbl)
        "Druckverhältnis" <- w383
        n198 = Subtract(x=w260, y=w259) -> (x-y=w393:dbl)
        n199 = Greater?(x=w393, y=1.0) -> (0:w267:bool)
        "Fl.Pumpe an" <- w267
        n200 = feedback #3() -> (w109:dbl)  [unwired: 1 in]
        n201 = Select(t=w109, s=w111, f=w103) -> (s? t:f=w110:dbl)
        n202 = feedback-in #3(w110) -> ()
        n203 = Less?(x=w265, y=60) -> (x < y?=w329:bool)
        "Temperatur Öl" <- w329
        n204 = Greater?(x=w383, y=1.5) -> (0:w381:bool)
        n205 = feedback #4(w103) -> (w104:dbl)
        n206 = Select(t=w103, s="Reset", f=w104) -> (s? t:f=w105:dbl)
        n207 = feedback-in #4(w105) -> ()
        n208 = Subtract(x=w103, y=w110) -> (x-y=w108:dbl)
        n209 = Subtract(x=w103, y=w105) -> (x-y=w107:dbl)
        n210 = expression code="x-3600"(w108) -> (w386:dbl)
        n211 = Build Array(w329, w381) -> (→"Warnungen":bool[])
        n212 = expression code="x-3600"(w107) -> (w388:dbl)
        n213 = Greater?(x=w108, y=720.0) -> (0:w268:bool)
        "Magnetventil" <- w268
        n214 = Build Array(w111, w268, w267) -> (→"Status Komponenten":bool[])
        n215 = call "Verdichternamen.vi"("Array"=w102) -> ("Dynamic Data"=w384:dynamicdata)  [unwired: 10 in]
        n216 = Seconds To Date/Time(time stamp (now)=w386) -> (date time rec=w330:T15)  [unwired: 1 in]
        n217 = Seconds To Date/Time(time stamp (now)=w388) -> (date time rec=w397:T15)  [unwired: 1 in]
        n218 = Unbundle By Name(w397) -> ("second"=w396:i32, "minute"=w395:i32, "hour"=w389:i32)
        n219 = Unbundle By Name(w330) -> ("second"=w399:i32, "minute"=w398:i32, "hour"=w387:i32)
        n220 = Bundle("second"=w399, "minute"=w398, "hour"=w387) -> (→"Verdichteraktivität":cluster{"second":i32, "minute":i32, "hour":i32})  [unwired: 1 in]
        n221 = Bundle("second"=w396, "minute"=w395, "hour"=w389) -> (→"Betriebszeit":cluster{"second":i32, "minute":i32, "hour":i32})  [unwired: 1 in]
        n222 = Merge Signals(w155, w154, w273, w384) -> (w292:dynamicdata)
        n223 = flat-sequence {
          tunnel: [w488] -> w407
          tunnel: [w487] -> w406
          tunnel: w310 -> [w486]
          tunnel: w309 -> [w485]
          tunnel: [w483] -> w306
          tunnel: "Identität!" -> [w482]
          tunnel: "Dateiname!" -> [w481]
          tunnel: "Speichern" -> [w480]
          tunnel: "tag" -> [w479]
          tunnel: w407 -> [w586]
          tunnel: w406 -> [w585]
          tunnel: [w581] -> w313
          tunnel: [w583] -> w312
          tunnel: w311 -> [w582]
          frame #0 {
            n224 = Index Array(array=w485) -> (element=w484:timestamp)  [unwired: 1 in]
            n225 = event shown="[1] \"Speichern\": Value Change" {
              selector: _ -> [_ _ _]
              dyn-events: _ -> [_ _ _]
              timeout: 5 -> [_ _ _]
              tunnel: [_ w498 _] -> w488
              tunnel: w486 -> [_ w493 _]
              tunnel: ["" w497 ""] -> w487
              tunnel: w484 -> [_ w496 w567]
              tunnel: [_ _ w565] -> w483
              tunnel: w482 -> [_ w495 _]
              tunnel: w481 -> [_ w494 _]
              tunnel: w480 -> [_ w492 _]
              tunnel: w479 -> [_ w491 _]
              event Timeout {
                n226 = event-data() -> ()  [unwired: 1 in, 1 out]
              }
              event "Speichern": Value Change {
                n227 = event-data() -> ()  [unwired: 1 in, 1 out]
                n228 = case shown="True" w492 {
                  tunnel: [w530 _] -> w498
                  tunnel: [w525 _] -> w497
                  tunnel: w496 -> [w517 _]
                  tunnel: w495 -> [w501 _]
                  tunnel: w494 -> [w513 _]
                  tunnel: w493 -> [w512 _]
                  tunnel: w491 -> [w500 _]
                  frame False {
                    w504 = "\r"
                    n229 = property on="Dateiname!" class="Str"("DisabledEnum"=T4."Disabled and Grayed Out" ("Disabled")) -> ()  [unwired: 2 in, 2 out]
                    n230 = for {
                      N: 1 -> [_]
                      tunnel: ["Zeit"] -> w510 mode=indexing
                      tunnel: ["Kommentar"] -> w506 mode=indexing
                    }
                    n231 = Format Date/Time String(time format string (%c)="%d-%m-%Y_%H.%M ", seconds (now)=w517) -> (date/time string=w518:string)  [unwired: 1 in]
                    n232 = Concatenate Strings(w501, "\\", w518, w513, ".lvm" ("string")) -> (w520:string)
                    n233 = Insert Into Array(array=w512, index (row)=0, new element=w510) -> (w508:string[][])  [unwired: 1 in]
                    n234 = Build Path(base path=path "\\\\pcift88\\Studenten/HT-Waermepumpe/Messdaten" ("file path (dialog if empty)"), name or relative path=w520) -> (appended path=w515:path)
                    n235 = Concatenate Strings(w501, "\t", "tag: " ("string"), w500) -> (w499:string)
                    n236 = Insert Into Array(array=w508, new element=w506) -> (w507:string[][])  [unwired: 2 in]
                    n237 = Open/Create/Replace File(file path (use dialog)=w515, operation (0:open)=T11."replace or create with confirmation") -> (refnum out=→"refnum out":refnum<file>, error out=w530:errorcluster)  [unwired: 4 in, 1 out]
                    n238 = Transpose 2D Array(2D array=w507) -> (transposed array=w528:string[][])
                    n239 = Format Date/Time String(seconds (now)=w517) -> (date/time string=w527:string)  [unwired: 2 in]
                    n240 = Strip Path(path=w515) -> (name=w514:string)  [unwired: 1 out]
                    n241 = Array To Spreadsheet String(array=w528, 3:"%s" ("format string")) -> (spreadsheet string=w526:string)  [unwired: 1 in]
                    n242 = Concatenate Strings(w499, w504, w504, w514, w504, w504, w527, w504, w504, w526, w504, w504) -> (w525:string)
                  }
                  frame True {
                    n243 = local read "refnum out"() -> (w534:refnum<file>)
                    n244 = property on="Dateiname!" class="Str"("DisabledEnum"=T4."Enabled" ("Disabled")) -> ()  [unwired: 2 in, 2 out]
                    n245 = Close File(refnum=w534) -> ()  [unwired: 1 in, 2 out]
                  }
                }
              }
              event "Comment": Value Change {
                # "Umlaute + ß ersetzen, quick&dirty 4.1.2016"
                n246 = event-data() -> ()  [unwired: 1 in, 1 out]
                n247 = flat-sequence {
                  tunnel: ["Kommentar"] -> w535
                  tunnel: w567 -> [w571]
                  frame #0 {
                    w573 = "\r"
                    n248 = local read "Historie"() -> (w575:string)
                    n249 = Get Date/Time String(seconds (now)=w571, want seconds? (F)=TRUE) -> (time string=w574:string)  [unwired: 1 in, 1 out]
                    n250 = Concatenate Strings(w575, w574, " -> ", "Kommentar", w573, w573) -> (→"Historie":string)
                  }
                  frame #1 {
                    n251 = local write "Kommentar"("") -> ()
                  }
                }
                n252 = Search and Replace String(replace all?=TRUE, input string=w535, search string="ä", replace string="ae") -> (result string=w557:string)  [unwired: 4 in, 3 out]
                n253 = Search and Replace String(replace all?=TRUE, input string=w557, search string="ü", replace string="ue") -> (result string=w556:string)  [unwired: 4 in, 3 out]
                n254 = Search and Replace String(replace all?=TRUE, input string=w556, search string="ö", replace string="oe") -> (result string=w555:string)  [unwired: 4 in, 3 out]
                n255 = Search and Replace String(replace all?=TRUE, input string=w555, search string="ß", replace string="ss") -> (result string=w536:string)  [unwired: 4 in, 3 out]
                n256 = Search and Replace String(replace all?=TRUE, input string=w536, search string="Ä", replace string="Ae") -> (result string=w545:string)  [unwired: 4 in, 3 out]
                n257 = Search and Replace String(replace all?=TRUE, input string=w545, search string="Ü", replace string="Ue") -> (result string=w544:string)  [unwired: 4 in, 3 out]
                n258 = Search and Replace String(replace all?=TRUE, input string=w544, search string="Ö", replace string="Oe") -> (result string=w537:string)  [unwired: 4 in, 3 out]
                n259 = for {
                  N: 1 -> [_]
                  tunnel: [w568] -> w565 mode=indexing
                  tunnel: w537 -> [w568]
                }
              }
            }
          }
          frame #1 {
            n260 = local read "refnum out"() -> (w578:refnum<file>)
            n261 = Concatenate Strings(w585, w582) -> (w584:string)
            n262 = Not A Number/Path/Refnum?(number/path/refnum=w578) -> (NaN/Path/Refnum?=w579:bool)
            n263 = Set File Position(refnum=w578, from (0:start)=enum16{"start", "end", "current"}."end", error in=w586) -> (refnum out=w587:refnum<file>, error out=w588:errorcluster)  [unwired: 1 in]
            n264 = Not(x=w579) -> (.not. x?=→"Speichert!":bool)
            n265 = Write to Text File(file (use dialog)=w587, text=w584, error in=w588) -> (refnum out=w581:refnum<file>, error out=w583:errorcluster)  [unwired: 1 in, 1 out]
          }
        }
        n266 = Empty String/Path?(string/path="Identität!") -> (empty?=w304:bool)
        n267 = Empty String/Path?(string/path="Dateiname!") -> (empty?=w303:bool)
        n268 = Or(x=w304, y=w303) -> (x .or. y?=w300:bool)
        n269 = call "Protokollordnung"("Signals"=w292) -> ("Signal Out"=w318:dynamicdata)  [unwired: 9 in, 1 out]
        n270 = Boolean To (0,1)(Boolean=w300) -> (0, 1=w301:i16)
        n271 = expression code="x*2"(w301) -> (w302:i16)
        n272 = property on="Speichern" class="Bool (strict)"("DisabledEnum"=w302) -> ()  [unwired: 2 in, 2 out]
        n273 = call "Convert from Dynamic Data"("Dynamic Data Type"=w318) -> ("Array of Waveform"=w319:waveform(dbl)[])  [unwired: 3 in]
        n274 = Array Size(array=w319) -> (size(s)=w296:i32)
        n275 = Concatenate Strings("%" ("string"), "." ("string"), ";%g" ("string")) -> (w321:string)
        n276 = Initialize Array(w321, w296) -> (w320:string[])
        n277 = for {
          tunnel: w319 -> [w592] mode=indexing
          tunnel: [w599] -> w316 mode=indexing
          tunnel: w320 -> [w597] mode=indexing
          tunnel: [w591] -> w310 mode=indexing
          tunnel: [w593] -> w309 mode=indexing
          tunnel: [w594] -> w315 mode=indexing
          n278 = Unbundle By Name(w592) -> ("Y"=w598:dbl[], "t0"=w590:timestamp)
          n279 = Get Waveform Attribute(5:w590, 6:"NI_ExpTimeStamp", 7:w592) -> (1:w593:timestamp)  [unwired: 1 in, 3 out]
          n280 = for {
            tunnel: w598 -> [w606] mode=indexing
            tunnel: [w605] -> w599 mode=indexing
            tunnel: w597 -> [w604]
            tunnel: w592 -> [w603]
            tunnel: [w602] -> w591 mode=indexing
            n281 = Format Into String(format string=w604, w606) -> (resulting string=w605:string)  [unwired: 2 in, 1 out]
            n282 = Get Waveform Attribute(5:"", 6:"NI_ChannelName", 7:w603) -> (1:w602:string)  [unwired: 1 in, 3 out]
          }
          n283 = Format Date/Time String(time format string (%c)="%H.%M.%S", seconds (now)=w593) -> (date/time string=w594:string)  [unwired: 1 in]
        }
        n284 = Insert Into Array(array=w316, index (row)=0, new element=w315) -> (w307:string[][])  [unwired: 1 in]
        n285 = Increment(x=w296) -> (x+1=w297:i32)
        n286 = Insert Into Array(array=w307, index (row)=w297, new element=w306) -> (w308:string[][])  [unwired: 1 in]
        n287 = Transpose 2D Array(2D array=w308) -> (transposed array=w305:string[][])
        n288 = Array To Spreadsheet String(array=w305, 3:"%s" ("format string")) -> (spreadsheet string=w311:string)  [unwired: 1 in]
      }
      frame #2 {
        n289 = Tick Count (ms)() -> (millisecond timer value=w724:u32)
        n290 = Subtract(x=w724, y=w723) -> (x-y=w722:u32)
        n291 = Divide(x=w722, y=1000.0) -> (x/y=→"Schleifendauer":dbl)
      }
    }
  }
  n292 = call <vilib>:"DAQmx Clear Task.vi"("task in"=w7, "error in"=w5) -> ()  [unwired: 13 in, 1 out]
  n293 = call <vilib>:"DAQmx Clear Task.vi"("task in"=w6, "error in"=w4) -> ()  [unwired: 13 in, 1 out]
  n294 = Close File(refnum=w32, error in=w31) -> (error out=w35:errorcluster)  [unwired: 1 out]
  n295 = call <vilib>:"General Error Handler.vi"("error in (no error)"=w35, "[exception action] (none:0)"=1 ("[exception code]"), "[exception code]"=1) -> ()  [unwired: 8 in, 5 out]
